vi "nirviAccSaturate16x16.vi"(1 "y":i16, 2 "x":i16) -> (0 "x+y":i16)   [LabVIEW 2020]
doc: "Computes the sum of two 16-bit numbers using saturation arithmetic to avoid integer overflow by returning a maximum or minimum value."
uses:
  <vilib>/rvi/Arithmetic/AddSubMult/XNode/nirviSatArithmetic.xnode
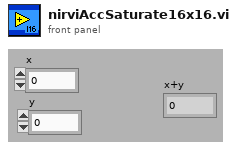
[diagram p1: front panel]
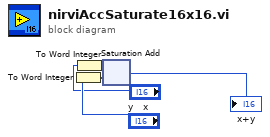
[diagram p0: block diagram]
diagram:
  n1 = To Word Integer(number="y") -> (16bit integer=w1:i16)
  n2 = To Word Integer(number="x") -> (16bit integer=w2:i16)
  n3 = xnode "Saturation Add"("x"=w2, "y"=w1) -> ("x+y"=→"x+y":i16)
